vi "3.3.vi"() -> ()   [LabVIEW 2019]
panel:
  out "Waveform Graph":dbl[](graph)
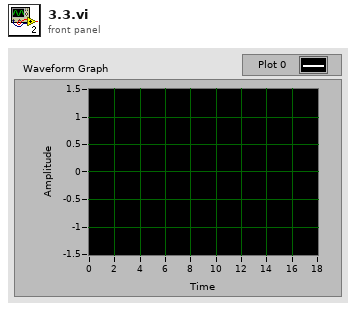
[diagram p1: front panel]
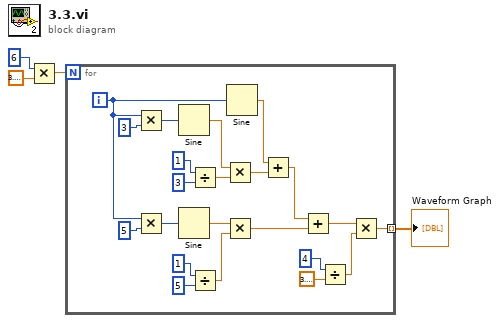
[diagram p0: block diagram]
diagram:
  n1 = Multiply(x=6, y=3.141592653589793) -> (x*y=w1:dbl)
  n2 = for {
    N: w1 -> [_]
    tunnel: [w5] -> w4 mode=indexing
    i -> [w15]
    n3 = Multiply(x=w15, y=3) -> (x*y=w25:i32)
    n4 = Multiply(x=w15, y=5) -> (x*y=w19:i32)
    n5 = Sine(x=w25) -> (sin(x)=w21:dbl)
    n6 = Sine(x=w19) -> (sin(x)=w16:dbl)
    n7 = Divide(x=1, y=3) -> (x/y=w22:dbl)
    n8 = Divide(x=1, y=5) -> (x/y=w17:dbl)
    n9 = Multiply(x=w21, y=w22) -> (x*y=w13:dbl)
    n10 = Multiply(x=w16, y=w17) -> (x*y=w12:dbl)
    n11 = Sine(x=w15) -> (sin(x)=w14:dbl)
    n12 = Add(x=w14, y=w13) -> (x+y=w11:dbl)
    n13 = Add(x=w11, y=w12) -> (x+y=w7:dbl)
    n14 = Divide(x=4, y=3.141592653589793) -> (x/y=w6:dbl)
    n15 = Multiply(x=w7, y=w6) -> (x*y=w5:dbl)
  }
  "Waveform Graph" <- w4
